vi "Configure Input Math.vi"(0 "VISA resource name":refnum<visa-resource-name>, 1 "Filter On/Off (F: Off)":bool, 2 "Points (2)":dbl=2.0 min=2.0 max=64.0 step=1.0, 3 "Window (1)":dbl=1.0 min=1.0 max=10.0 step=1.0, 5 "Input (0: A)":u16(ring) items=["A", "B"], 6 "Min/Max Source (0: Kelvin)":u16(ring) items=["Kelvin", "Celsius", "Sensor Units", "Linear Data"], 7 "Equation (0: y=mx+b)":u16(ring) items=["y=mx+b", "y=m(x+b)"], 9 "Variable M Value (1.0000)":dbl=1.0 min=-1000.0 max=1000.0 step=0.0001 format="%.4f", 11 "error in (no error)":errorcluster, 12 "Variable B Value (0.0000)":dbl min=-100000000.0 max=100000000.0 step=0.0001 format="%.4f", 13 "X Source (0: Kelvin)":u16(ring) items=["Kelvin", "Celsius", "Sensor Units"], 14 "B Source (0: Variable B Value)":u16(ring) items=["Variable B Value", "+Setpoint 1", "-Setpoint 1", "+Setpoint 2", "-Setpoint 2"]) -> (4 "VISA resource name out":refnum<visa-resource-name>, 15 "error out":errorcluster)   [LabVIEW 2013, in "Lake Shore Cryotronics 331.lvlib"]
doc: "This VI configures the math functions for the 331 inputs. Linear Equation, Min/Max, and Filter are all configured with this vi."
uses:
  Lake Shore Cryotronics 331.lvlib
panel:
  # "Linear Equation"
  # "Min/Max"
  # "Filter"
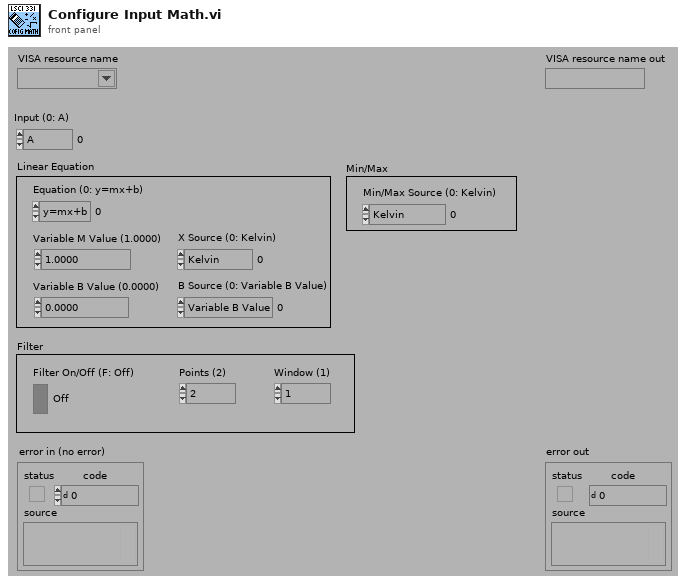
[diagram p1: front panel]
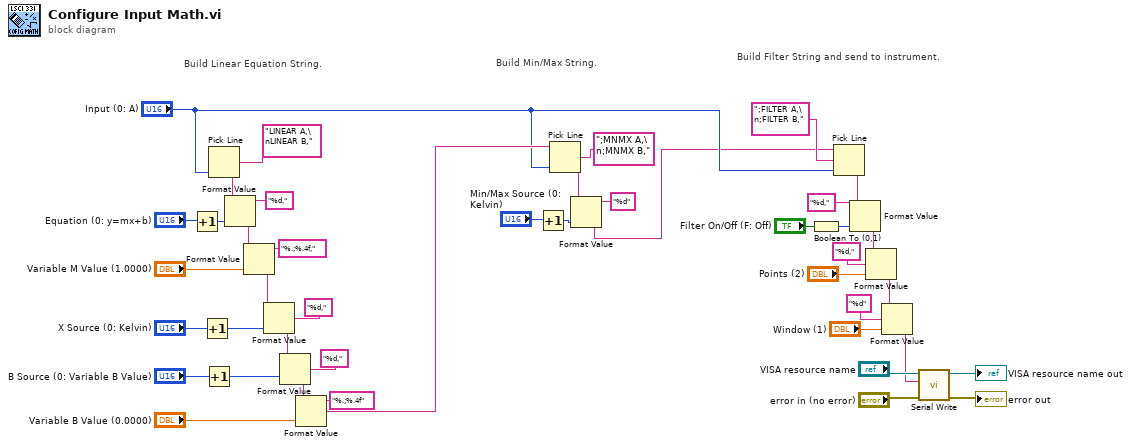
[diagram p0: block diagram]
diagram:
  # "Build Filter String and send to instrument."
  # "Build Min/Max String."
  # "Build Linear Equation String."
  n1 = Increment(x="Equation (0: y=mx+b)") -> (x+1=w27:u16)
  n2 = Increment(x="X Source (0: Kelvin)") -> (x+1=w38:u16)
  n3 = Increment(x="B Source (0: Variable B Value)") -> (x+1=w33:u16)
  n4 = Pick Line(multi-line string="LINEAR A,\nLINEAR B,", line index="Input (0: A)") -> (output string=w28:string)  [unwired: 1 in]
  n5 = Format Value(string ("")=w28, format string="%d,", value (0)=w27) -> (output string=w31:string)
  n6 = Format Value(string ("")=w31, format string="%.;%.4f,", value (0)="Variable M Value (1.0000)") -> (output string=w39:string)
  n7 = Format Value(string ("")=w39, format string="%d,", value (0)=w38) -> (output string=w40:string)
  n8 = Format Value(string ("")=w40, format string="%d,", value (0)=w33) -> (output string=w43:string)
  n9 = Format Value(string ("")=w43, format string="%.;%.4f", value (0)="Variable B Value (0.0000)") -> (output string=w20:string)
  n10 = Increment(x="Min/Max Source (0: Kelvin)") -> (x+1=w24:u16)
  n11 = Pick Line(string ("")=w20, multi-line string=";MNMX A,\n;MNMX B,", line index="Input (0: A)") -> (output string=w23:string)
  n12 = Format Value(string ("")=w23, format string="%d", value (0)=w24) -> (output string=w1:string)
  n13 = Boolean To (0,1)(Boolean="Filter On/Off (F: Off)") -> (0, 1=w16:i16)
  n14 = Pick Line(string ("")=w1, multi-line string=";FILTER A,\n;FILTER B,", line index="Input (0: A)") -> (output string=w15:string)
  n15 = Format Value(string ("")=w15, format string="%d,", value (0)=w16) -> (output string=w14:string)
  n16 = Format Value(string ("")=w14, format string="%d,", value (0)="Points (2)") -> (output string=w9:string)
  n17 = Format Value(string ("")=w9, format string="%d", value (0)="Window (1)") -> (output string=w4:string)
  n18 = call "Serial Write.vi"("error in (no error)"="error in (no error)", "Write Buffer (\"\")"=w4, "VISA resource name"="VISA resource name") -> ("error out"=→"error out":errorcluster, "VISA resource name out"=→"VISA resource name out":refnum<visa-resource-name>)  [unwired: 6 in, 1 out]
